vi "Delete_unwanted_rows.vi"(1 "Selected Rows":i32[](array[numeric]), 2 "Filename":path) -> ()   [LabVIEW 2010]
uses:
  Globals/Constants_global.vi
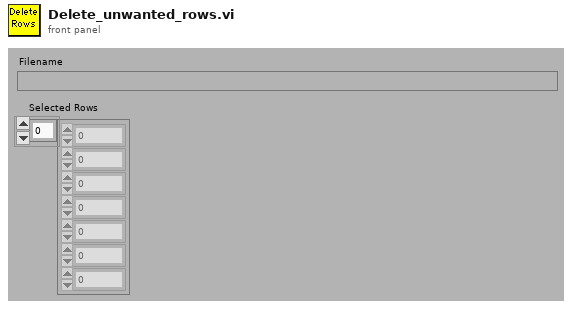
[diagram p1: front panel]
types:
  T1 = enum16{"read/write", "read-only", "write-only", "write-only (truncate)"}
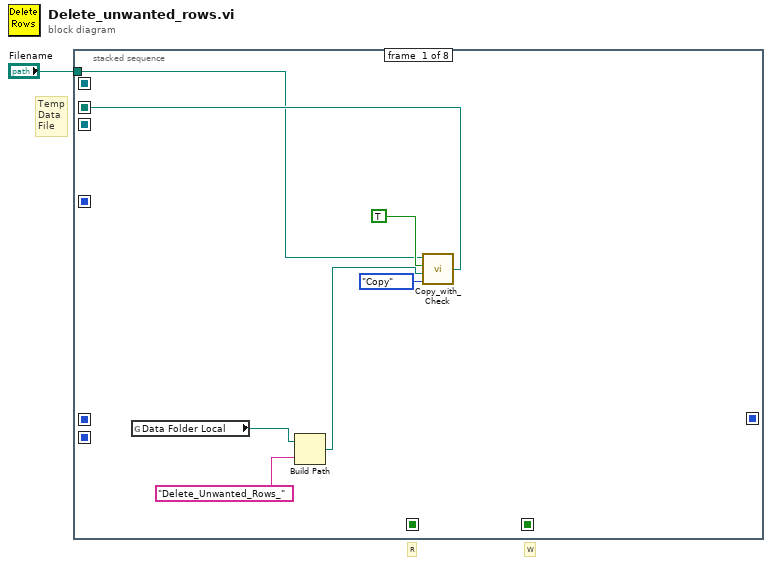
[diagram p0: block diagram]
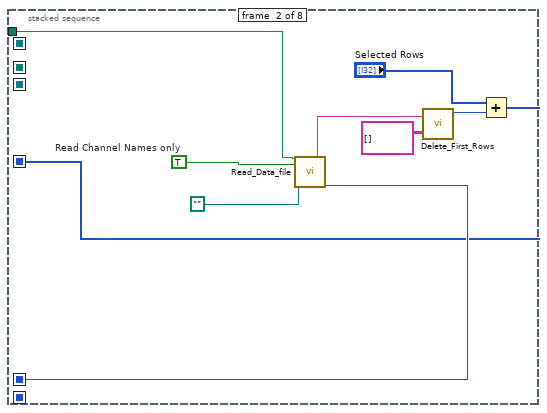
[diagram p2: hidden frame]
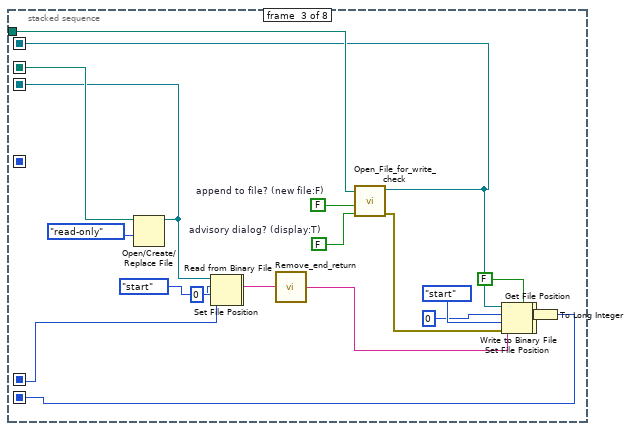
[diagram p3: hidden frame]
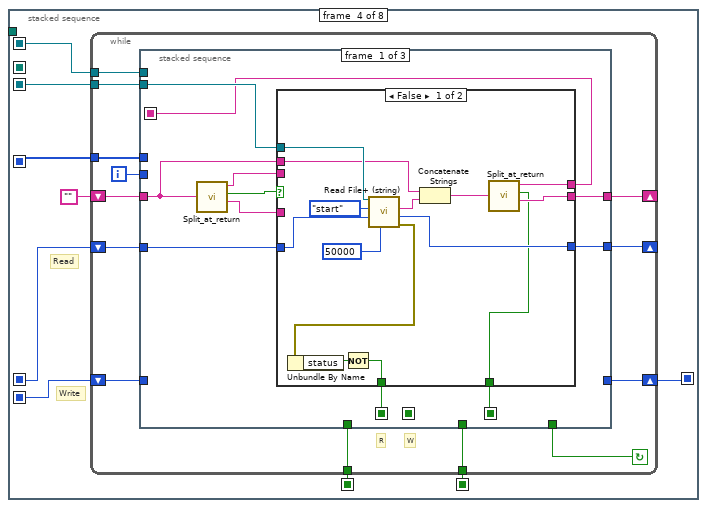
[diagram p4: hidden frame]
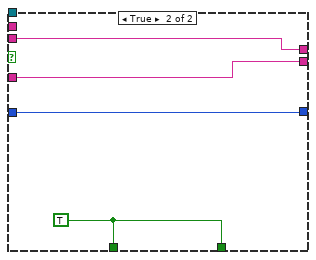
[diagram p5: hidden frame]
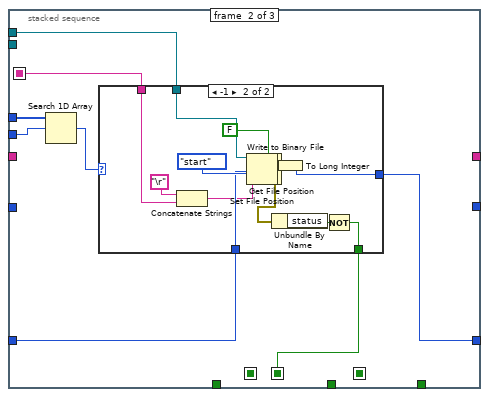
[diagram p6: hidden frame]
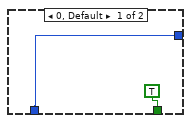
[diagram p7: hidden frame]
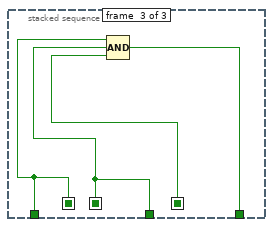
[diagram p8: hidden frame]
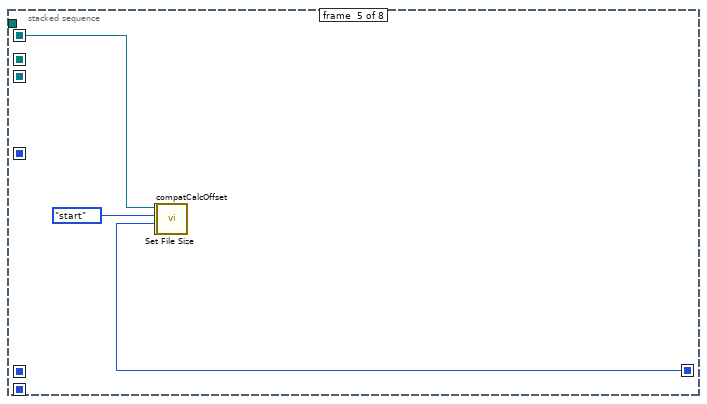
[diagram p9: hidden frame]
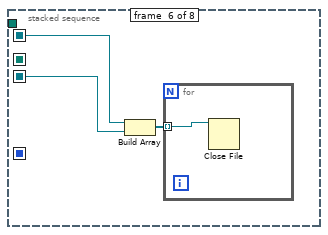
[diagram p10: hidden frame]
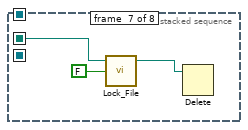
[diagram p11: hidden frame]
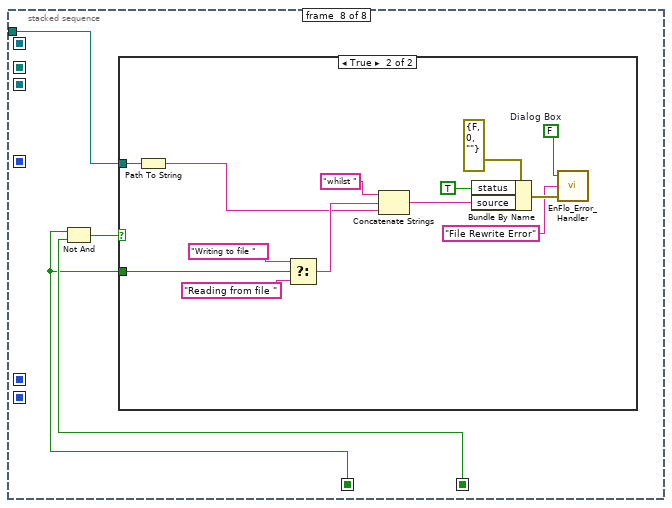
[diagram p12: hidden frame]
diagram:
  # "W"
  # "R"
  # "Temp\nData\nFile"
  n1 = stacked-sequence {
    seq-local: [w5 _ _ _ _ _ _ _] -> [_ _ w37 _ _ _ w135 _]
    seq-local: [_ _ w32 _ _ _ _ _] -> [_ _ _ w49 _ w130 _ _]
    seq-local: [_ _ w30 _ _ _ _ _] -> [_ _ _ w48 w128 w131 _ _]
    seq-local: [_ w14 _ _ _ _ _ _] -> [_ _ w31 w43 _ _ _ _]
    seq-local: [_ _ _ w47 _ _ _ _] -> [_ _ _ _ _ _ _ w137]
    seq-local: [_ _ _ w46 _ _ _ _] -> [_ _ _ _ _ _ _ w139]
    seq-local: [_ _ _ w45 _ _ _ _] -> [_ _ _ _ w127 _ _ _]
    seq-local: [_ w9 _ _ _ _ _ _] -> [_ _ _ w44 _ _ _ _]
    seq-local: [_ _ w26 _ _ _ _ _] -> [_ _ _ w42 _ _ _ _]
    tunnel: "Filename" -> [w4 w15 w38 _ _ _ _ w136]
    frame #0 {
      n2 = global read "Constants_global.vi" "Data Folder Local"() -> (w7:path)
      n3 = Build Path(base path=w7, name or relative path="Delete_Unwanted_Rows_") -> (appended path=w3:path)
      n4 = call "Copy_with_Check.vi"("Mode"=enum16{"Move", "Copy"}."Copy", "Target Path"=w3, "Variable Target?"=TRUE, "Source Path"=w4) -> ("Pathname Out"=w5:path)
    }
    frame #1 {
      w16 = TRUE  # Read Channel Names only
      n5 = call "Read_Data_file.vi"("Results file"=w15, "Read Channel Names only"=w16, "Template File"=path "") -> ("Filetype"=w13:string, "mark after read (chars.)"=w14:i32)  [unwired: 2 in, 13 out]
      n6 = call "Delete_First_Rows.vi"("Data In"=string[][] [], "File Type"=w13) -> ("Rows removed"=w12:i32)  [unwired: 1 out]
      n7 = Add(x="Selected Rows", y=w12) -> (x+y=w9:i32[])
    }
    frame #2 {
      w39 = FALSE  # advisory dialog? (display:T)
      w40 = FALSE  # append to file? (new file:F)
      n8 = Open/Create/Replace File(file path (use dialog)=w37, access (0:read/write)=T1."read-only" ("open mode (0)")) -> (refnum out=w32:refnum<file>)  [unwired: 1 in, 5 out]
      n9 = Set File Position(offset (in bytes) (0)=0 ("pos offset (0)"), refnum=w32, from (0:start)=enum16{"start", "end", "current"}."start" ("pos mode (rel. to current:2)")) -> (refnum out=w25:refnum<file>, error out=w24:errorcluster)  [unwired: 1 in]
      n10 = Read from Binary File(8:w24, 10:w31, 11:w25) -> (2:w28:string)  [unwired: 6 out]
      n11 = call "Remove_end_return.vi"("Input string"=w28) -> ("Output string"=w27:string)
      n12 = call "Open_File_for_write_check.vi"("advisory dialog? (display:T)"=w39, "append to file? (new file:F)"=w40, "file path"=w38) -> ("error out"=w29:errorcluster, "refnum"=w30:refnum<file>)  [unwired: 7 out]
      n13 = Set File Position(offset (in bytes) (0)=0 ("pos offset (0)"), refnum=w30, from (0:start)=enum16{"start", "end", "current"}."start" ("pos mode (0:2)"), error in=w29) -> (refnum out=w23:refnum<file>, error out=w22:errorcluster)
      n14 = Write to Binary File(file (use dialog)=w23, data=w27, error in=w22, 5:FALSE ("prepend array or string size? (T)")) -> (refnum out=w21:refnum<file>, error out=w20:errorcluster)  [unwired: 3 out]
      n15 = Get File Position(4:w20, 7:w21) -> (2:w19:i64)  [unwired: 2 out]
      n16 = To Long Integer(number=w19) -> (32bit integer=w26:i32)
    }
    frame #3 {
      # "Write"
      # "Read"
      n17 = while {
        tunnel: [w53] -> w46
        tunnel: [w54] -> w47
        tunnel: w48 -> [w57]
        shift-left: w42 -> [w58]
        shift-right: [w56] -> w45
        tunnel: w49 -> [w60]
        shift-left: w43 -> [w62]
        shift-right: [w61] -> _
        shift-left: "" -> [w63]
        shift-right: [w59] -> _
        tunnel: w44 -> [w52]
        i -> [w51]
        stop <- w55 continue-if-true
        # "R"
        # "W"
        n18 = stacked-sequence {
          seq-local: [w66 _ _] -> [_ w97 _]
          seq-local: [_ w93 _] -> [_ _ w119]
          seq-local: [w67 _ _] -> [_ _ w121]
          seq-local: [w68 _ _] -> [_ _ w120]
          tunnel: w63 -> [w71 _ _]
          tunnel: w62 -> [w74 _ _]
          tunnel: [w73 _ _] -> w61
          tunnel: w60 -> [w72 _ _]
          tunnel: [w70 _ _] -> w59
          tunnel: w58 -> [_ w100 _]
          tunnel: w57 -> [_ w99 _]
          tunnel: [_ w98 _] -> w56
          tunnel: [_ _ w122] -> w55
          tunnel: [_ _ w120] -> w54
          tunnel: [_ _ w119] -> w53
          tunnel: w52 -> [_ w96 _]
          tunnel: w51 -> [_ w95 _]
          frame #0 {
            n19 = call "Split_at_return.vi"("String"=w71) -> ("before substring"=w65:string, "Matched?"=w64:bool, "after substring"=w69:string)  [unwired: 1 in, 1 out]
            n20 = case shown="False" w64 {
              tunnel: w74 -> [w88 w92]
              tunnel: [w86 w92] -> w73
              tunnel: w72 -> [w85 _]
              tunnel: w71 -> [w83 _]
              tunnel: [w81 w91] -> w70
              tunnel: w69 -> [_ w91]
              tunnel: [w78 w90] -> w68
              tunnel: [w76 w90] -> w67
              tunnel: [w77 w89] -> w66
              tunnel: w65 -> [_ w89]
              frame False {
                n21 = call <vilib>:"Read File+ (string).vi"("count"=50000, "pos offset (bytes:0)"=w88, "pos mode (rel. to current:2)"=enum16{"start", "end", "current"}."start", "refnum"=w85) -> ("error out"=w80:errorcluster, "mark after read (bytes)"=w86:i32, "string"=w84:string)  [unwired: 1 in, 4 out]
                n22 = Unbundle By Name(w80) -> ("status"=w79:bool)
                n23 = Not(x=w79) -> (.not. x?=w78:bool)
                n24 = Concatenate Strings(w83, w84) -> (w82:string)
                n25 = call "Split_at_return.vi"("String"=w82) -> ("before substring"=w77:string, "Matched?"=w76:bool, "after substring"=w81:string)  [unwired: 1 in, 1 out]
              }
              frame True {
                w90 = TRUE
              }
            }
          }
          frame #1 {
            n26 = Search 1D Array(1D array=w96, element=w95) -> (index of element=w94:i32)  [unwired: 1 out]
            n27 = case shown="-1" w94 {
              tunnel: w100 -> [w102 w117]
              tunnel: w99 -> [_ w116]
              tunnel: [w102 w109] -> w98
              tunnel: w97 -> [_ w114]
              tunnel: [TRUE w110] -> w93
              frame 0, Default {
              }
              frame -1 {
                n28 = Concatenate Strings("\r", w114) -> (w113:string)
                n29 = Set File Position(offset (in bytes) (0)=w117, refnum=w116, from (0:start)=enum16{"start", "end", "current"}."start" ("pos mode (0:2)")) -> (refnum out=w108:refnum<file>, error out=w107:errorcluster)  [unwired: 1 in]
                n30 = Write to Binary File(file (use dialog)=w108, data=w113, error in=w107, 5:FALSE ("prepend array or string size? (T)")) -> (refnum out=w106:refnum<file>, error out=w105:errorcluster)  [unwired: 3 out]
                n31 = Get File Position(4:w105, 7:w106) -> (0:w111:errorcluster, 2:w104:i64)  [unwired: 1 out]
                n32 = Unbundle By Name(w111) -> ("status"=w112:bool)
                n33 = To Long Integer(number=w104) -> (32bit integer=w109:i32)
                n34 = Not(x=w112) -> (.not. x?=w110:bool)
              }
            }
          }
          frame #2 {
            n35 = Compound Arithmetic op=AND(w120, w119, w121) -> (w122:bool)
          }
        }
      }
    }
    frame #4 {
      n36 = call <vilib>:"compatCalcOffset.vi"("pos offset (0)"=w127, "pos mode (0:1)"=enum16{"start", "end", "current"}."start", "refnum"=w128) -> ("error out"=w125:errorcluster, "offset"=w124:i32, "dup refnum"=w123:refnum<file>)  [unwired: 1 in, 5 out]
      n37 = Set File Size(4:w125, 6:w124, 7:w123) -> ()  [unwired: 2 out]
    }
    frame #5 {
      n38 = Build Array(w131, w130) -> (w129:refnum<file>[])
      n39 = for {
        tunnel: w129 -> [w132] mode=indexing
        n40 = Close File(refnum=w132) -> ()  [unwired: 1 in, 2 out]
      }
    }
    frame #6 {
      n41 = call "Lock_File.vi"("Lock File"=FALSE, "path"=w135) -> ("dup path"=w134:path)  [unwired: 1 in, 2 out]
      n42 = Delete(path (use dialog)=w134) -> ()  [unwired: 1 in, 6 out]
    }
    frame #7 {
      n43 = Not And(1:w139, 2:w137) -> (0:w138:bool)
      n44 = case shown="True" w138 {
        tunnel: w137 -> [_ w152]
        tunnel: w136 -> [_ w142]
        frame False {
        }
        frame True {
          w145 = FALSE  # Dialog Box
          n45 = Path To String(path=w142) -> (string=w141:string)
          n46 = Select(t="Writing to file ", s=w152, f="Reading from file ") -> (s? t:f=w148:string)
          n47 = Concatenate Strings("whilst ", w148, w141) -> (w143:string)
          n48 = Bundle By Name(cluster=errorcluster {"status"=FALSE, "code"=0, "source"=""} ("error in (no error)"), "status"=TRUE ("Bundle Element"), "source"=w143) -> (w146:errorcluster)
          n49 = call "EnFlo_Error_Handler.vi"("error in (no error)"=w146, "Error Type"="File Rewrite Error", "Dialog Box (T)"=w145) -> ()  [unwired: 3 out]
        }
      }
    }
  }
